vi "Excel Data Log 2.vi"(4 "Channel Settings":T9={"Supply Voltage [Vdc]"=14.4, "Max Supply Current [Idc]"=50.0, "Settling Delay"=10.0, "Temp Criteria"=0.0, "Voltage Steps [Vrms]"=[], "User Notes"="", "Config Wave File Path"=path "", "Config Voltage [Vrms]"=0.1, "Channel Configuration List"={"Channel Configuration Cluster"={"Input"=enum."1 AVG", "Enable"=TRUE, "User Notes"="1", "Voltage Range"=15.0, "Current Range"=2.5}, "Channel Configuration Cluster 2"={"Input"=enum."1 AVG", "Enable"=TRUE, "User Notes"="2", "Voltage Range"=15.0, "Current Range"=2.5}, "Channel Configuration Cluster 3"={"Input"=enum."1 AVG", "Enable"=TRUE, "User Notes"="3", "Voltage Range"=15.0, "Current Range"=2.5}, "Channel Configuration Cluster 4"={"Input"=enum."1 AVG", "Enable"=TRUE, "User Notes"="4", "Voltage Range"=15.0, "Current Range"=2.5}, "Channel Configuration Cluster 5"={"Input"=enum."1", "Enable"=TRUE, "User Notes"="5", "Voltage Range"=15.0, "Current Range"=2.5}, "Channel Configuration Cluster 6"={"Input"=enum."1", "Enable"=TRUE, "User Notes"="6", "Voltage Range"=15.0, "Current Range"=2.5}, "Channel Configuration Cluster 7"={"Input"=enum."1", "Enable"=TRUE, "User Notes"="7", "Voltage Range"=15.0, "Current Range"=2.5}, "Channel Configuration Cluster 8"={"Input"=enum."1", "Enable"=TRUE, "User Notes"="8", "Voltage Range"=15.0, "Current Range"=2.5}, "Channel Configuration Cluster 9"={"Input"=enum."1", "Enable"=TRUE, "User Notes"="9", "Voltage Range"=15.0, "Current Range"=2.5}, "Channel Configuration Cluster 10"={"Input"=enum."2 AVG", "Enable"=TRUE, "User Notes"="10", "Voltage Range"=15.0, "Current Range"=2.5}, "Channel Configuration Cluster 11"={"Input"=enum."2 AVG", "Enable"=TRUE, "User Notes"="11", "Voltage Range"=15.0, "Current Range"=2.5}, "Channel Configuration Cluster 12"={"Input"=enum."2 AVG", "Enable"=TRUE, "User Notes"="12", "Voltage Range"=15.0, "Current Range"=2.5}, "Channel Configuration Cluster 13"={"Input"=enum."2 AVG", "Enable"=TRUE, "User Notes"="13", "Voltage Range"=15.0, "Current Range"=2.5}, "Channel Configuration Cluster 14"={"Input"=enum."2", "Enable"=TRUE, "User Notes"="14", "Voltage Range"=15.0, "Current Range"=2.5}, "Channel Configuration Cluster 15"={"Input"=enum."2", "Enable"=TRUE, "User Notes"="15", "Voltage Range"=15.0, "Current Range"=2.5}, "Channel Configuration Cluster 16"={"Input"=enum."2", "Enable"=TRUE, "User Notes"="16", "Voltage Range"=15.0, "Current Range"=2.5}, "Channel Configuration Cluster 17"={"Input"=enum."2", "Enable"=TRUE, "User Notes"="17", "Voltage Range"=15.0, "Current Range"=2.5}}, "User Gains"={"Gain 1"=12.0, "Gain 2"=11.9, "Gain 3"=0.0, "Gain 4"=0.0, "Gain 5"=0.0, "Gain 6"=0.0}, "Gains"={"Gain 1"=11.908530403349321, "Gain 2"=11.85949105887029, "Gain 3"=0.0, "Gain 4"=0.0, "Gain 5"=0.0, "Gain 6"=0.0}, "Gain Array"={"Gain 1"=11.948064032758305, "Gain 2"=11.797736859280617, "Gain 3"=11.962639910718805, "Gain 4"=11.924703126556764, "Gain 5"=11.642892109168656, "Gain 6"=11.458169944769443, "Gain 7"=11.65709969408898, "Gain 8"=11.754705913936172, "Gain 9"=11.848154878633066, "Gain 10"=11.818689497840571, "Gain 11"=11.899914309524277, "Gain 12"=11.77881456393431, "Gain 13"=11.93961179471489, "Gain 14"=11.746688316913492, "Gain 15"=11.861889454079613, "Gain 16"=11.852640030144613, "Gain 17"=11.690623229258875}, "Wave File Path 1"=path "C:/Users/gm8988/Desktop/Data Log", "Wave File Path 2"=path "", "Wave File Path 3"=path "", "Wave File Path 4"=path "", "Range"=FALSE, "CF"=FALSE} {"Gain Array"."Gain 17" format="%.2f"; "Gain Array"."Gain 16" format="%.2f"; "Gain Array"."Gain 15" format="%.2f"; "Gain Array"."Gain 14" format="%.2f"; "Gain Array"."Gain 13" format="%.2f"; "Gain Array"."Gain 12" format="%.2f"; "Gain Array"."Gain 11" format="%.2f"; "Gain Array"."Gain 10" format="%.2f"; "Gain Array"."Gain 9" format="%.2f"; "Gain Array"."Gain 8" format="%.2f"; "Gain Array"."Gain 7" format="%.2f"; "Gain Array"."Gain 6" format="%.2f"; "Gain Array"."Gain 5" format="%.2f"; "Gain Array"."Gain 4" format="%.2f"; "Gain Array"."Gain 3" format="%.2f"; "Gain Array"."Gain 2" format="%.2f"; "Gain Array"."Gain 1" format="%.2f"; "Gains"."Gain 6" format="%.2f"; "Gains"."Gain 5" format="%.2f"; "Gains"."Gain 4" format="%.2f"; "Gains"."Gain 3" format="%.2f"; "Gains"."Gain 2" format="%.2f"; "Gains"."Gain 1" format="%.2f"; "User Gains"."Gain 6" format="%.2f"; "User Gains"."Gain 5" format="%.2f"; "User Gains"."Gain 4" format="%.2f"; "User Gains"."Gain 3" format="%.2f"; "User Gains"."Gain 2" format="%.2f"; "User Gains"."Gain 1" format="%.2f"; "Channel Configuration List"."Channel Configuration Cluster 17"."Current Range" items=["1 <500m>"=0.5, "2 <1>"=1.0, "5 <2.5>"=2.5, "10 <5>"=5.0, "20 <10>"=10.0, "50 <25>"=25.0]; "Channel Configuration List"."Channel Configuration Cluster 17"."Voltage Range" items=["1.5 <0.75>"=0.75, "3 <1.5>"=1.5, "6 <3>"=3.0, "10 <5>"=5.0, "15 <7.5>"=7.5, "30 <15>"=15.0, "60 <30>"=30.0, "100 <50>"=50.0, "150 <75>"=75.0, "300 <150>"=150.0, "600 <300>"=300.0, "1000 <500>"=500.0]; "Channel Configuration List"."Channel Configuration Cluster 16"."Current Range" items=["1 <500m>"=0.5, "2 <1>"=1.0, "5 <2.5>"=2.5, "10 <5>"=5.0, "20 <10>"=10.0, "50 <25>"=25.0]; "Channel Configuration List"."Channel Configuration Cluster 16"."Voltage Range" items=["1.5 <0.75>"=0.75, "3 <1.5>"=1.5, "6 <3>"=3.0, "10 <5>"=5.0, "15 <7.5>"=7.5, "30 <15>"=15.0, "60 <30>"=30.0, "100 <50>"=50.0, "150 <75>"=75.0, "300 <150>"=150.0, "600 <300>"=300.0, "1000 <500>"=500.0]; "Channel Configuration List"."Channel Configuration Cluster 15"."Current Range" items=["1 <500m>"=0.5, "2 <1>"=1.0, "5 <2.5>"=2.5, "10 <5>"=5.0, "20 <10>"=10.0, "50 <25>"=25.0]; "Channel Configuration List"."Channel Configuration Cluster 15"."Voltage Range" items=["1.5 <0.75>"=0.75, "3 <1.5>"=1.5, "6 <3>"=3.0, "10 <5>"=5.0, "15 <7.5>"=7.5, "30 <15>"=15.0, "60 <30>"=30.0, "100 <50>"=50.0, "150 <75>"=75.0, "300 <150>"=150.0, "600 <300>"=300.0, "1000 <500>"=500.0]; "Channel Configuration List"."Channel Configuration Cluster 14"."Current Range" items=["1 <500m>"=0.5, "2 <1>"=1.0, "5 <2.5>"=2.5, "10 <5>"=5.0, "20 <10>"=10.0, "50 <25>"=25.0]; "Channel Configuration List"."Channel Configuration Cluster 14"."Voltage Range" items=["1.5 <0.75>"=0.75, "3 <1.5>"=1.5, "6 <3>"=3.0, "10 <5>"=5.0, "15 <7.5>"=7.5, "30 <15>"=15.0, "60 <30>"=30.0, "100 <50>"=50.0, "150 <75>"=75.0, "300 <150>"=150.0, "600 <300>"=300.0, "1000 <500>"=500.0]; "Channel Configuration List"."Channel Configuration Cluster 13"."Current Range" items=["1 <500m>"=0.5, "2 <1>"=1.0, "5 <2.5>"=2.5, "10 <5>"=5.0, "20 <10>"=10.0, "50 <25>"=25.0]; "Channel Configuration List"."Channel Configuration Cluster 13"."Voltage Range" items=["1.5 <0.75>"=0.75, "3 <1.5>"=1.5, "6 <3>"=3.0, "10 <5>"=5.0, "15 <7.5>"=7.5, "30 <15>"=15.0, "60 <30>"=30.0, "100 <50>"=50.0, "150 <75>"=75.0, "300 <150>"=150.0, "600 <300>"=300.0, "1000 <500>"=500.0]; "Channel Configuration List"."Channel Configuration Cluster 12"."Current Range" items=["1 <500m>"=0.5, "2 <1>"=1.0, "5 <2.5>"=2.5, "10 <5>"=5.0, "20 <10>"=10.0, "50 <25>"=25.0]; "Channel Configuration List"."Channel Configuration Cluster 12"."Voltage Range" items=["1.5 <0.75>"=0.75, "3 <1.5>"=1.5, "6 <3>"=3.0, "10 <5>"=5.0, "15 <7.5>"=7.5, "30 <15>"=15.0, "60 <30>"=30.0, "100 <50>"=50.0, "150 <75>"=75.0, "300 <150>"=150.0, "600 <300>"=300.0, "1000 <500>"=500.0]; "Channel Configuration List"."Channel Configuration Cluster 11"."Current Range" items=["1 <500m>"=0.5, "2 <1>"=1.0, "5 <2.5>"=2.5, "10 <5>"=5.0, "20 <10>"=10.0, "50 <25>"=25.0]; "Channel Configuration List"."Channel Configuration Cluster 11"."Voltage Range" items=["1.5 <0.75>"=0.75, "3 <1.5>"=1.5, "6 <3>"=3.0, "10 <5>"=5.0, "15 <7.5>"=7.5, "30 <15>"=15.0, "60 <30>"=30.0, "100 <50>"=50.0, "150 <75>"=75.0, "300 <150>"=150.0, "600 <300>"=300.0, "1000 <500>"=500.0]; "Channel Configuration List"."Channel Configuration Cluster 10"."Current Range" items=["1 <500m>"=0.5, "2 <1>"=1.0, "5 <2.5>"=2.5, "10 <5>"=5.0, "20 <10>"=10.0, "50 <25>"=25.0]; "Channel Configuration List"."Channel Configuration Cluster 10"."Voltage Range" items=["1.5 <0.75>"=0.75, "3 <1.5>"=1.5, "6 <3>"=3.0, "10 <5>"=5.0, "15 <7.5>"=7.5, "30 <15>"=15.0, "60 <30>"=30.0, "100 <50>"=50.0, "150 <75>"=75.0, "300 <150>"=150.0, "600 <300>"=300.0, "1000 <500>"=500.0]; "Channel Configuration List"."Channel Configuration Cluster 9"."Voltage Range" items=["1.5 <0.75>"=0.75, "3 <1.5>"=1.5, "6 <3>"=3.0, "10 <5>"=5.0, "15 <7.5>"=7.5, "30 <15>"=15.0, "60 <30>"=30.0, "100 <50>"=50.0, "150 <75>"=75.0, "300 <150>"=150.0, "600 <300>"=300.0, "1000 <500>"=500.0]; "Channel Configuration List"."Channel Configuration Cluster 9"."Current Range" items=["10m <5m>"=0.005, "20m <10m>"=0.01, "50m <25m>"=0.025, "100m <50m>"=0.05, "200m <100m>"=0.1, "500m <250m>"=0.25, "1 <500m>"=0.5, "2 <1>"=1.0, "5 <2.5>"=2.5]; "Channel Configuration List"."Channel Configuration Cluster 8"."Voltage Range" items=["1.5 <0.75>"=0.75, "3 <1.5>"=1.5, "6 <3>"=3.0, "10 <5>"=5.0, "15 <7.5>"=7.5, "30 <15>"=15.0, "60 <30>"=30.0, "100 <50>"=50.0, "150 <75>"=75.0, "300 <150>"=150.0, "600 <300>"=300.0, "1000 <500>"=500.0]; "Channel Configuration List"."Channel Configuration Cluster 8"."Current Range" items=["10m <5m>"=0.005, "20m <10m>"=0.01, "50m <25m>"=0.025, "100m <50m>"=0.05, "200m <100m>"=0.1, "500m <250m>"=0.25, "1 <500m>"=0.5, "2 <1>"=1.0, "5 <2.5>"=2.5]; "Channel Configuration List"."Channel Configuration Cluster 7"."Voltage Range" items=["1.5 <0.75>"=0.75, "3 <1.5>"=1.5, "6 <3>"=3.0, "10 <5>"=5.0, "15 <7.5>"=7.5, "30 <15>"=15.0, "60 <30>"=30.0, "100 <50>"=50.0, "150 <75>"=75.0, "300 <150>"=150.0, "600 <300>"=300.0, "1000 <500>"=500.0]; "Channel Configuration List"."Channel Configuration Cluster 7"."Current Range" items=["10m <5m>"=0.005, "20m <10m>"=0.01, "50m <25m>"=0.025, "100m <50m>"=0.05, "200m <100m>"=0.1, "500m <250m>"=0.25, "1 <500m>"=0.5, "2 <1>"=1.0, "5 <2.5>"=2.5]; "Channel Configuration List"."Channel Configuration Cluster 6"."Voltage Range" items=["1.5 <0.75>"=0.75, "3 <1.5>"=1.5, "6 <3>"=3.0, "10 <5>"=5.0, "15 <7.5>"=7.5, "30 <15>"=15.0, "60 <30>"=30.0, "100 <50>"=50.0, "150 <75>"=75.0, "300 <150>"=150.0, "600 <300>"=300.0, "1000 <500>"=500.0]; "Channel Configuration List"."Channel Configuration Cluster 6"."Current Range" items=["10m <5m>"=0.005, "20m <10m>"=0.01, "50m <25m>"=0.025, "100m <50m>"=0.05, "200m <100m>"=0.1, "500m <250m>"=0.25, "1 <500m>"=0.5, "2 <1>"=1.0, "5 <2.5>"=2.5]; "Channel Configuration List"."Channel Configuration Cluster 5"."Voltage Range" items=["1.5 <0.75>"=0.75, "3 <1.5>"=1.5, "6 <3>"=3.0, "10 <5>"=5.0, "15 <7.5>"=7.5, "30 <15>"=15.0, "60 <30>"=30.0, "100 <50>"=50.0, "150 <75>"=75.0, "300 <150>"=150.0, "600 <300>"=300.0, "1000 <500>"=500.0]; "Channel Configuration List"."Channel Configuration Cluster 5"."Current Range" items=["10m <5m>"=0.005, "20m <10m>"=0.01, "50m <25m>"=0.025, "100m <50m>"=0.05, "200m <100m>"=0.1, "500m <250m>"=0.25, "1 <500m>"=0.5, "2 <1>"=1.0, "5 <2.5>"=2.5]; "Channel Configuration List"."Channel Configuration Cluster 4"."Voltage Range" items=["1.5 <0.75>"=0.75, "3 <1.5>"=1.5, "6 <3>"=3.0, "10 <5>"=5.0, "15 <7.5>"=7.5, "30 <15>"=15.0, "60 <30>"=30.0, "100 <50>"=50.0, "150 <75>"=75.0, "300 <150>"=150.0, "600 <300>"=300.0, "1000 <500>"=500.0]; "Channel Configuration List"."Channel Configuration Cluster 4"."Current Range" items=["10m <5m>"=0.005, "20m <10m>"=0.01, "50m <25m>"=0.025, "100m <50m>"=0.05, "200m <100m>"=0.1, "500m <250m>"=0.25, "1 <500m>"=0.5, "2 <1>"=1.0, "5 <2.5>"=2.5]; "Channel Configuration List"."Channel Configuration Cluster 3"."Voltage Range" items=["1.5 <0.75>"=0.75, "3 <1.5>"=1.5, "6 <3>"=3.0, "10 <5>"=5.0, "15 <7.5>"=7.5, "30 <15>"=15.0, "60 <30>"=30.0, "100 <50>"=50.0, "150 <75>"=75.0, "300 <150>"=150.0, "600 <300>"=300.0, "1000 <500>"=500.0]; "Channel Configuration List"."Channel Configuration Cluster 3"."Current Range" items=["10m <5m>"=0.005, "20m <10m>"=0.01, "50m <25m>"=0.025, "100m <50m>"=0.05, "200m <100m>"=0.1, "500m <250m>"=0.25, "1 <500m>"=0.5, "2 <1>"=1.0, "5 <2.5>"=2.5]; "Channel Configuration List"."Channel Configuration Cluster 2"."Voltage Range" items=["1.5 <0.75>"=0.75, "3 <1.5>"=1.5, "6 <3>"=3.0, "10 <5>"=5.0, "15 <7.5>"=7.5, "30 <15>"=15.0, "60 <30>"=30.0, "100 <50>"=50.0, "150 <75>"=75.0, "300 <150>"=150.0, "600 <300>"=300.0, "1000 <500>"=500.0]; "Channel Configuration List"."Channel Configuration Cluster 2"."Current Range" items=["10m <5m>"=0.005, "20m <10m>"=0.01, "50m <25m>"=0.025, "100m <50m>"=0.05, "200m <100m>"=0.1, "500m <250m>"=0.25, "1 <500m>"=0.5, "2 <1>"=1.0, "5 <2.5>"=2.5]; "Channel Configuration List"."Channel Configuration Cluster"."Voltage Range" items=["1.5 <0.75>"=0.75, "3 <1.5>"=1.5, "6 <3>"=3.0, "10 <5>"=5.0, "15 <7.5>"=7.5, "30 <15>"=15.0, "60 <30>"=30.0, "100 <50>"=50.0, "150 <75>"=75.0, "300 <150>"=150.0, "600 <300>"=300.0, "1000 <500>"=500.0]; "Channel Configuration List"."Channel Configuration Cluster"."Current Range" items=["10m <5m>"=0.005, "20m <10m>"=0.01, "50m <25m>"=0.025, "100m <50m>"=0.05, "200m <100m>"=0.1, "500m <250m>"=0.25, "1 <500m>"=0.5, "2 <1>"=1.0, "5 <2.5>"=2.5]; "Settling Delay" min=0.0 format="%<%H:%M:%S>t"}, 5 "JPEG2 Path":path, 6 "Cancel":bool, 7 "JPEG1 Path":path, 8 "error in":errorcluster, 10 "Datalog Cluster Array":T1 {"WT1800 Averages"."Vrms" format="%.3f"; "WT1800 Averages"."Irms" format="%.3f"; "WT1800 Averages"."Power" format="%.3f"; "WT1800 Averages"."Vpkpk" format="%.3f"; "WT1800 Averages"."Ipkpk" format="%.3f"; "WT1800 Measurements"."Vrms" format="%.3f"; "WT1800 Measurements"."Irms" format="%.3f"; "WT1800 Measurements"."Power" format="%.3f"; "WT1800 Measurements"."Vpkpk" format="%.3f"; "WT1800 Measurements"."Ipkpk" format="%.3f"; "DSA Averages"."Vrms" format="%.3f"; "DSA Averages"."Vdc" format="%.3f"; "DSA Averages"."Vpk+" format="%.3f"; "DSA Averages"."Vpk-" format="%.3f"; "DSA Averages"."Vpkpk" format="%.3f"; "DSA Measurements"."Vrms" format="%.3f"; "DSA Measurements"."Vdc" format="%.3f"; "DSA Measurements"."Vpk+" format="%.3f"; "DSA Measurements"."Vpk-" format="%.3f"; "DSA Measurements"."Vpkpk" format="%.3f"}, 11 "Template Path":path) -> (0 "error out":errorcluster)   [LabVIEW 2021]
uses:
  Datalog Controls/Select_Data.ctl
  Controls/Settings Control.ctl
  Controls/Channel Configuration List.ctl
  Controls/Channel Configuration Cluster.ctl
  Controls/Channel Configuration Cluster High Current.ctl
  Controls/Gain Averages.ctl
  Controls/Gain Array.ctl
  Controls/Datalog Cluster Array.ctl
  Controls/Datalog Bundle Control.ctl
  Controls/WT1800 Functions.ctl
  Controls/WT1800 Measurements.ctl
  Controls/WT1800 Readings.ctl
  Controls/DSA Functions.ctl
  Controls/DSA Measurements.ctl
  Controls/DSA Readings.ctl
  Datalog Controls/States.ctl
  Datalog Controls/Data.ctl
  <vilib>/Utility/NIReport.llb/NI_report.lvclass
  <vilib>/Utility/miscctls.llb/LVPointTypeDef.ctl
  <vilib>/Utility/error.llb/DialogType.ctl
panel:
  out "Time Taken (Seconds)":u32
  in  "Generate":bool
  in  "Manual Select":bool
  in  "Select All":bool=TRUE
  in  "Select Data":T15={"Vrms Data"=TRUE, "Vpkpk Data"=TRUE, "Irms Data"=TRUE, "Power Data"=TRUE, "Ipkpk Data"=TRUE, "Temp Data"=TRUE}
  in  "Detailed Report":bool=TRUE
  in  "Stop":bool
  in  "Summary Report":bool
  # "Ver 1.2.1"
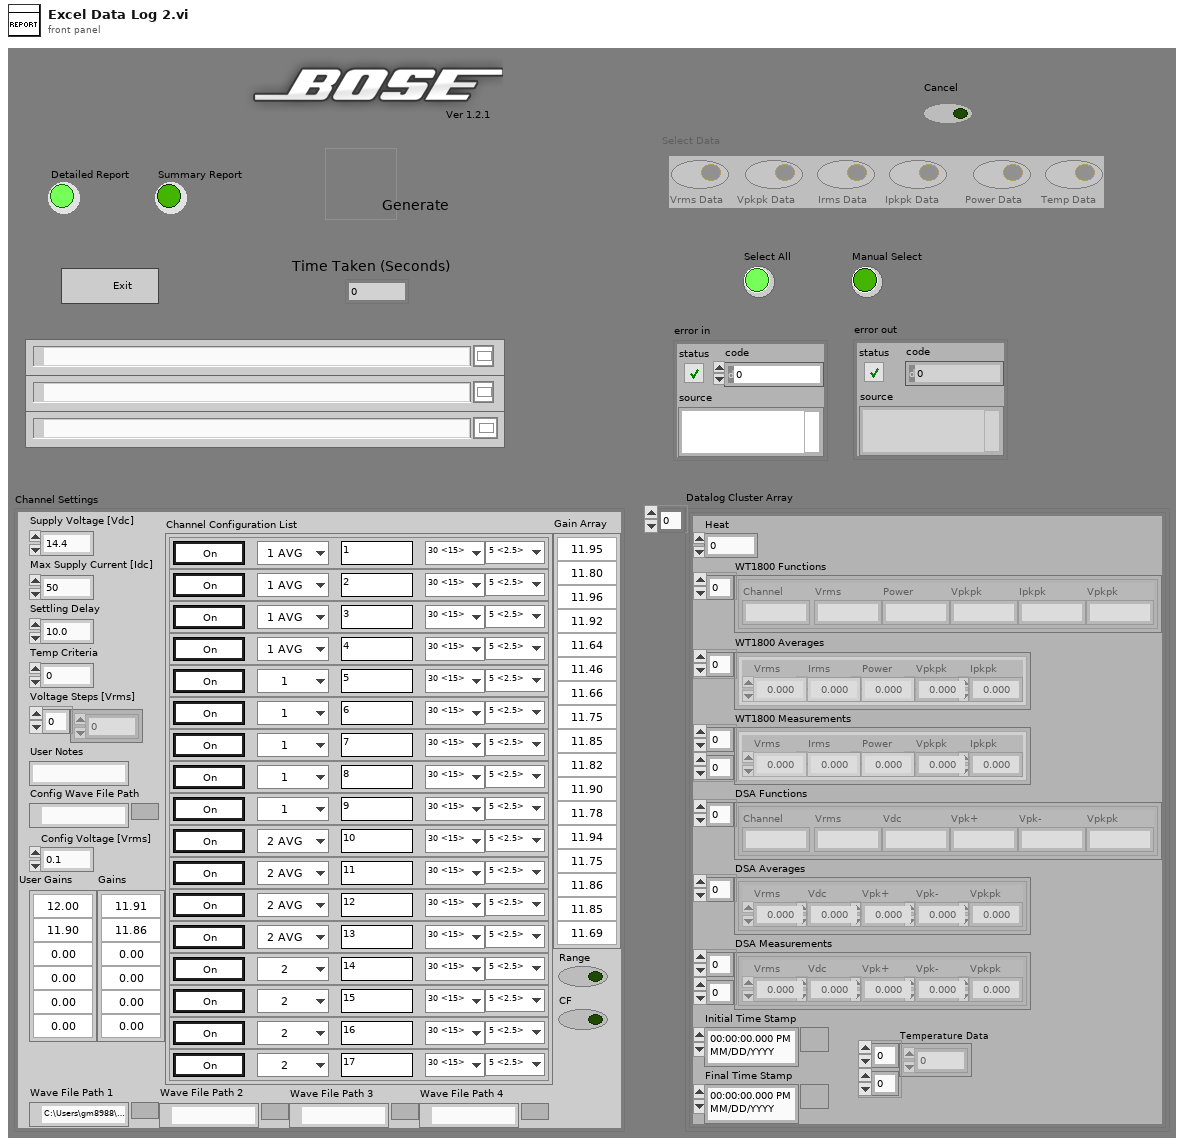
[diagram p1: front panel]
types:
  T1 = typedef "Datalog Cluster Array.ctl" = T2[]
  T2 = typedef "Datalog Bundle Control.ctl" = cluster{"Heat":dbl, "WT1800 Functions":T3, "WT1800 Averages":T4, "WT1800 Measurements":T5[][], "DSA Functions":T6, "DSA Averages":T7, "DSA Measurements":T8[][], "Initial Time Stamp":timestamp, "Final Time Stamp":timestamp, "Temperature Data":sgl[][]}
  T3 = typedef "WT1800 Functions.ctl" = cluster{"Channel":string, "Vrms":string, "Power":string, "Vpkpk":string, "Ipkpk":string, "Vpkpk":string}[]
  T4 = typedef "WT1800 Measurements.ctl" = T5[]
  T5 = typedef "WT1800 Readings.ctl" = cluster{"Vrms":sgl, "Irms":sgl, "Power":sgl, "Vpkpk":sgl, "Ipkpk":sgl}
  T6 = typedef "DSA Functions.ctl" = cluster{"Channel":string, "Vrms":string, "Vdc":string, "Vpk+":string, "Vpk-":string, "Vpkpk":string}[]
  T7 = typedef "DSA Measurements.ctl" = T8[]
  T8 = typedef "DSA Readings.ctl" = cluster{"Vrms":sgl, "Vdc":sgl, "Vpk+":sgl, "Vpk-":sgl, "Vpkpk":sgl}
  T9 = typedef "Settings Control.ctl" = cluster{"Supply Voltage [Vdc]":sgl, "Max Supply Current [Idc]":sgl, "Settling Delay":dbl, "Temp Criteria":sgl, "Voltage Steps [Vrms]":sgl[], "User Notes":string, "Config Wave File Path":path, "Config Voltage [Vrms]":sgl, "Channel Configuration List":T10, "User Gains":T13, "Gains":T13, "Gain Array":T14, "Wave File Path 1":path, "Wave File Path 2":path, "Wave File Path 3":path, "Wave File Path 4":path, "Range":bool, "CF":bool}
  T10 = typedef "Channel Configuration List.ctl" = cluster{"Channel Configuration Cluster":T11, "Channel Configuration Cluster 2":T11, "Channel Configuration Cluster 3":T11, "Channel Configuration Cluster 4":T11, "Channel Configuration Cluster 5":T11, "Channel Configuration Cluster 6":T11, "Channel Configuration Cluster 7":T11, "Channel Configuration Cluster 8":T11, "Channel Configuration Cluster 9":T11, "Channel Configuration Cluster 10":T12, "Channel Configuration Cluster 11":T12, "Channel Configuration Cluster 12":T12, "Channel Configuration Cluster 13":T12, "Channel Configuration Cluster 14":T12, "Channel Configuration Cluster 15":T12, "Channel Configuration Cluster 16":T12, "Channel Configuration Cluster 17":T12}
  T11 = typedef "Channel Configuration Cluster.ctl" = cluster{"Input":enum16{"---", "1", "1 AVG", "2", "2 AVG", "3", "3 AVG", "4", "4 AVG"}, "Enable":bool, "User Notes":string, "Voltage Range":dbl, "Current Range":dbl}
  T12 = typedef "Channel Configuration Cluster High Current.ctl" = cluster{"Input":enum16{"---", "1", "1 AVG", "2", "2 AVG", "3", "3 AVG", "4", "4 AVG"}, "Enable":bool, "User Notes":string, "Voltage Range":dbl, "Current Range":dbl}
  T13 = typedef "Gain Averages.ctl" = cluster{"Gain 1":dbl, "Gain 2":dbl, "Gain 3":dbl, "Gain 4":dbl, "Gain 5":dbl, "Gain 6":dbl}
  T14 = typedef "Gain Array.ctl" = cluster{"Gain 1":dbl, "Gain 2":dbl, "Gain 3":dbl, "Gain 4":dbl, "Gain 5":dbl, "Gain 6":dbl, "Gain 7":dbl, "Gain 8":dbl, "Gain 9":dbl, "Gain 10":dbl, "Gain 11":dbl, "Gain 12":dbl, "Gain 13":dbl, "Gain 14":dbl, "Gain 15":dbl, "Gain 16":dbl, "Gain 17":dbl}
  T15 = typedef "Select_Data.ctl" = cluster{"Vrms Data":bool, "Vpkpk Data":bool, "Irms Data":bool, "Power Data":bool, "Ipkpk Data":bool, "Temp Data":bool}
  T16 = typedef "Data.ctl" = cluster{"Input Data 1D":T1, "Channel Settings":T9, "Select Data":T15, "Detailed Report ?":bool, "Path Settings:":cluster{"Template Path ":path, "Report Path":path, "JPEG1 Path ":path, "JPEG2 Path":path}, "Vrms_Sheet":string[][], "Irms_Sheet":string[][], "Power_Sheet":string[][], "Vpk_Sheet":string[][], "Ipk_Sheet":string[][], "Vrms_Avg":string[][], "Irms_Avg":string[][], "Power_Avg":string[][], "Vpk_Avg":string[][], "Ipk_Avg":string[][], "Report_Ref":refnum<class "NI_report.lvclass">, "User Name":string, "Temp_Sheet":string[][]}
  T17 = typedef "States.ctl" = enum16{"Initialize", "Poll", "Generate Report", "Error", "Exit"}
  T18 = typedef "LVPointTypeDef.ctl" = cluster{"Horizontal":i16, "Vertical":i16}
  T19 = enum8{"Enabled", "Disabled", "Disabled and Grayed Out"}
  T20 = typedef "DialogType.ctl" = u16
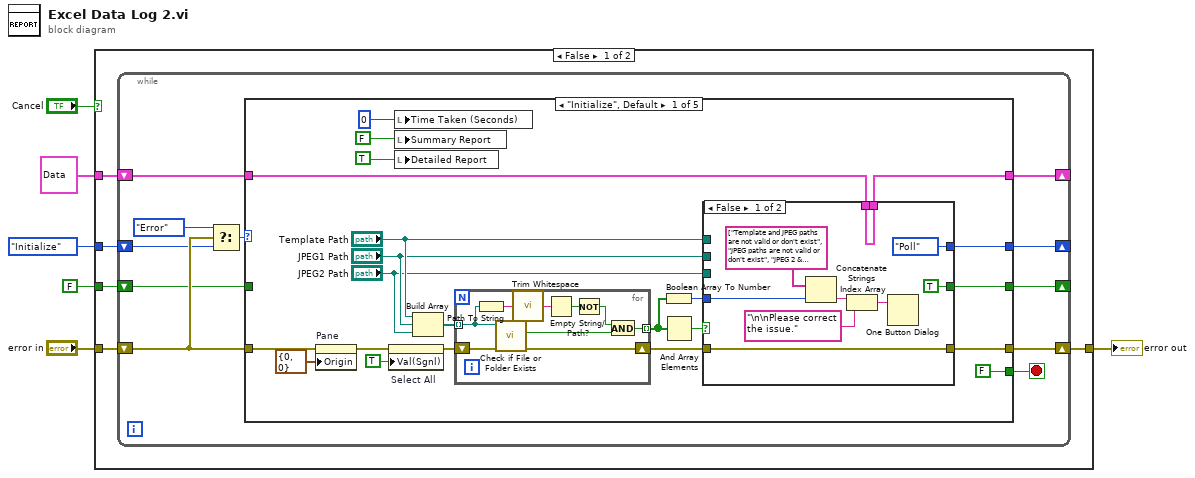
[diagram p0: block diagram]
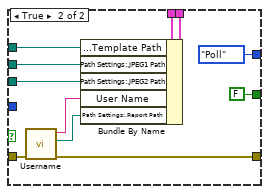
[diagram p2: hidden frame]
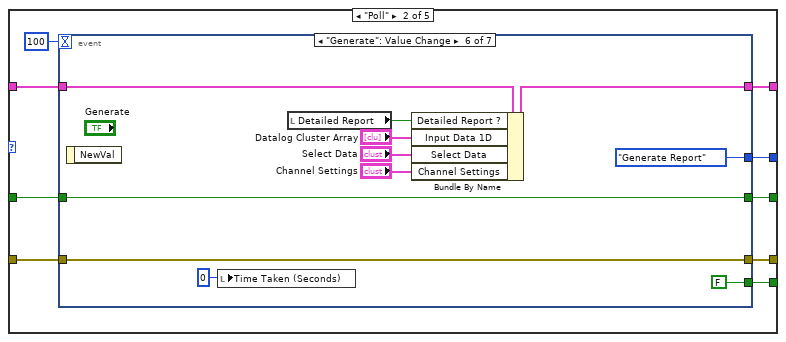
[diagram p3: hidden frame]
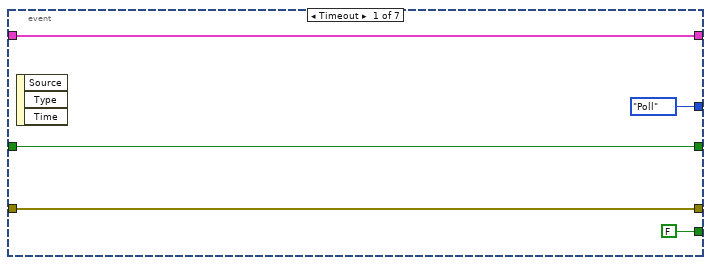
[diagram p4: hidden frame]
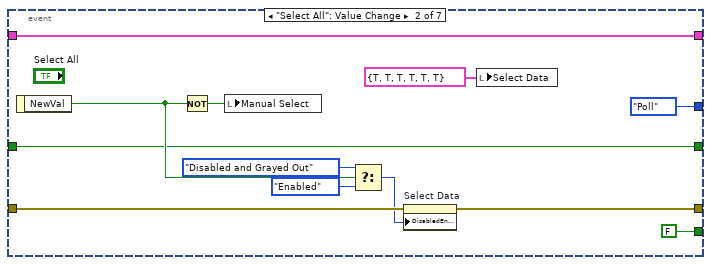
[diagram p5: hidden frame]
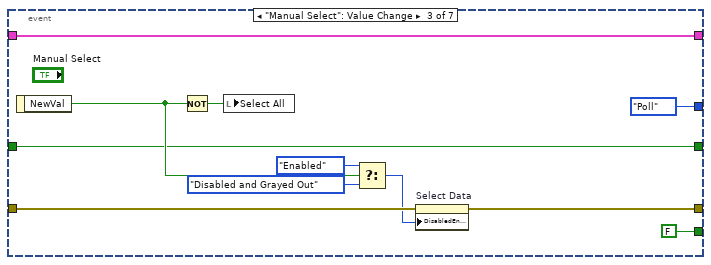
[diagram p6: hidden frame]
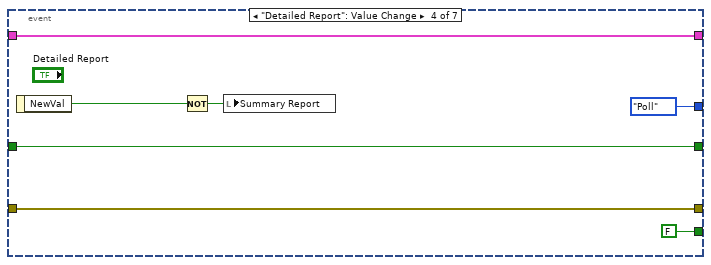
[diagram p7: hidden frame]
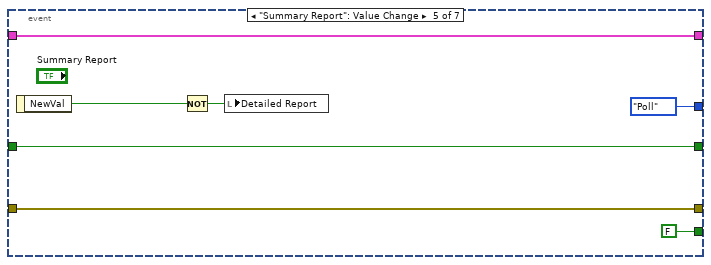
[diagram p8: hidden frame]
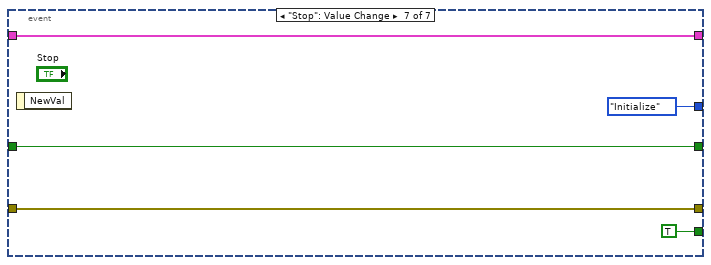
[diagram p9: hidden frame]
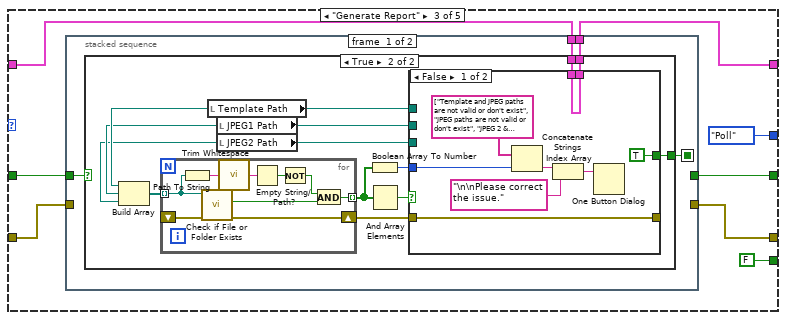
[diagram p10: hidden frame]
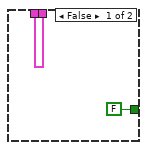
[diagram p11: hidden frame]
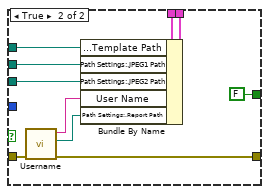
[diagram p12: hidden frame]
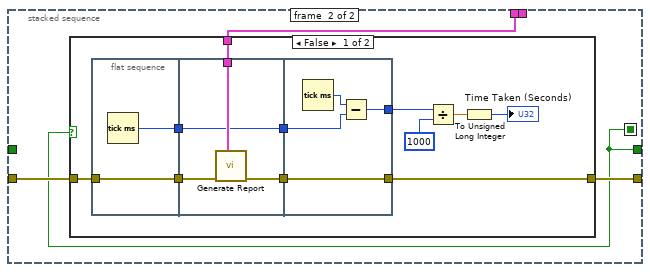
[diagram p13: hidden frame]
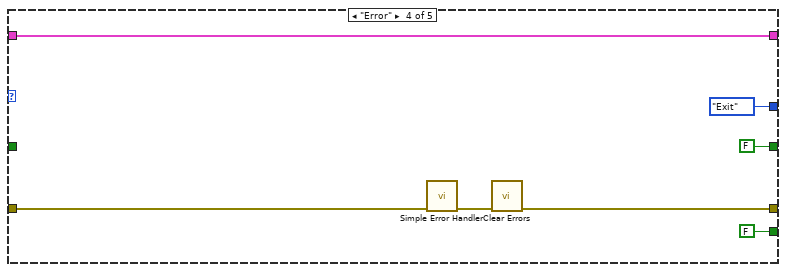
[diagram p15: hidden frame]
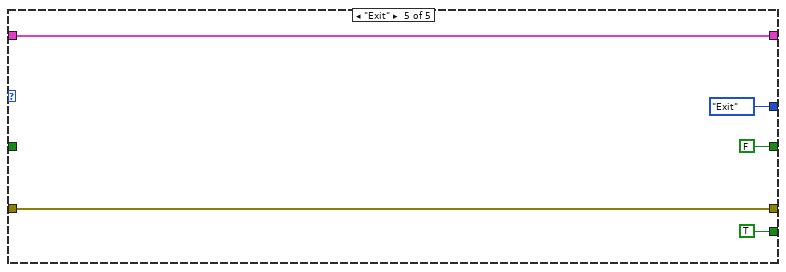
[diagram p16: hidden frame]
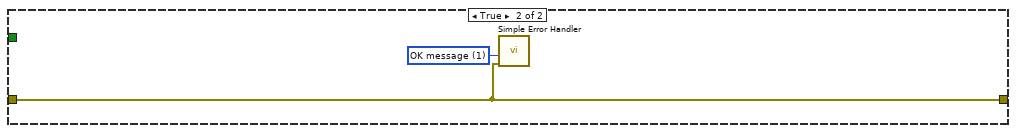
[diagram p17: hidden frame]
diagram:
  n1 = case shown="False" "Cancel" {
    tunnel: States."Initialize" -> [w11 _]
    tunnel: T16 {"Input Data 1D"=[], "Channel Settings"={"Supply Voltage [Vdc]"=0.0, "Max Supply Current [Idc]"=0.0, "Settling Delay"=0.0, "Temp Criteria"=0.0, "Voltage Steps [Vrms]"=[0.0, 0.25, 0.5, 1.0, 1.95, 3.0, 3.9, 5.5], "User Notes"="", "Config Wave File Path"=path "C:/ASD Power Point Beta 32J/Waveforms/150HzSine5Second.wav", "Config Voltage [Vrms]"=0.0, "Channel Configuration List"={"Channel Configuration Cluster"={"Input"=enum."---", "Enable"=FALSE, "User Notes"="", "Voltage Range"=0.0, "Current Range"=2.5}, "Channel Configuration Cluster 2"={"Input"=enum."---", "Enable"=FALSE, "User Notes"="", "Voltage Range"=0.0, "Current Range"=2.5}, "Channel Configuration Cluster 3"={"Input"=enum."---", "Enable"=FALSE, "User Notes"="", "Voltage Range"=0.0, "Current Range"=2.5}, "Channel Configuration Cluster 4"={"Input"=enum."---", "Enable"=FALSE, "User Notes"="", "Voltage Range"=0.0, "Current Range"=2.5}, "Channel Configuration Cluster 5"={"Input"=enum."---", "Enable"=FALSE, "User Notes"="", "Voltage Range"=0.0, "Current Range"=2.5}, "Channel Configuration Cluster 6"={"Input"=enum."---", "Enable"=FALSE, "User Notes"="", "Voltage Range"=0.0, "Current Range"=2.5}, "Channel Configuration Cluster 7"={"Input"=enum."---", "Enable"=FALSE, "User Notes"="", "Voltage Range"=0.0, "Current Range"=2.5}, "Channel Configuration Cluster 8"={"Input"=enum."---", "Enable"=FALSE, "User Notes"="", "Voltage Range"=0.0, "Current Range"=2.5}, "Channel Configuration Cluster 9"={"Input"=enum."---", "Enable"=FALSE, "User Notes"="", "Voltage Range"=0.0, "Current Range"=2.5}, "Channel Configuration Cluster 10"={"Input"=enum."---", "Enable"=FALSE, "User Notes"="", "Voltage Range"=0.0, "Current Range"=2.5}, "Channel Configuration Cluster 11"={"Input"=enum."---", "Enable"=FALSE, "User Notes"="", "Voltage Range"=0.0, "Current Range"=2.5}, "Channel Configuration Cluster 12"={"Input"=enum."---", "Enable"=FALSE, "User Notes"="", "Voltage Range"=0.0, "Current Range"=2.5}, "Channel Configuration Cluster 13"={"Input"=enum."---", "Enable"=FALSE, "User Notes"="", "Voltage Range"=0.0, "Current Range"=2.5}, "Channel Configuration Cluster 14"={"Input"=enum."---", "Enable"=FALSE, "User Notes"="", "Voltage Range"=0.0, "Current Range"=2.5}, "Channel Configuration Cluster 15"={"Input"=enum."---", "Enable"=FALSE, "User Notes"="", "Voltage Range"=0.0, "Current Range"=2.5}, "Channel Configuration Cluster 16"={"Input"=enum."---", "Enable"=FALSE, "User Notes"="", "Voltage Range"=0.0, "Current Range"=2.5}, "Channel Configuration Cluster 17"={"Input"=enum."---", "Enable"=FALSE, "User Notes"="", "Voltage Range"=0.0, "Current Range"=2.5}}, "User Gains"={"Gain 1"=0.0, "Gain 2"=0.0, "Gain 3"=0.0, "Gain 4"=0.0, "Gain 5"=0.0, "Gain 6"=0.0}, "Gains"={"Gain 1"=0.0, "Gain 2"=0.0, "Gain 3"=0.0, "Gain 4"=0.0, "Gain 5"=0.0, "Gain 6"=0.0}, "Gain Array"={"Gain 1"=0.0, "Gain 2"=0.0, "Gain 3"=0.0, "Gain 4"=0.0, "Gain 5"=0.0, "Gain 6"=0.0, "Gain 7"=0.0, "Gain 8"=0.0, "Gain 9"=0.0, "Gain 10"=0.0, "Gain 11"=0.0, "Gain 12"=0.0, "Gain 13"=0.0, "Gain 14"=0.0, "Gain 15"=0.0, "Gain 16"=0.0, "Gain 17"=0.0}, "Wave File Path 1"=path "", "Wave File Path 2"=path "", "Wave File Path 3"=path "", "Wave File Path 4"=path "", "Range"=FALSE, "CF"=FALSE}, "Select Data"={"Vrms Data"=FALSE, "Vpkpk Data"=FALSE, "Irms Data"=FALSE, "Power Data"=FALSE, "Ipkpk Data"=FALSE, "Temp Data"=FALSE}, "Detailed Report ?"=FALSE, "Path Settings:"={"Template Path "=path "E:/L&T Projects/Bose ASD/Excel Template/ASD Template.xltx", "Report Path"=path "E:/L&T Projects/Bose ASD/excel Reports", "JPEG1 Path "=path "C:/Users/Public/Pictures/Sample Pictures/Hydrangeas.jpg", "JPEG2 Path"=path "C:/Users/Public/Pictures/Sample Pictures/Lighthouse.jpg"}, "Vrms_Sheet"=[], "Irms_Sheet"=[], "Power_Sheet"=[], "Vpk_Sheet"=[], "Ipk_Sheet"=[], "Vrms_Avg"=[], "Irms_Avg"=[], "Power_Avg"=[], "Vpk_Avg"=[], "Ipk_Avg"=[], "Report_Ref"=refnum, "User Name"="", "Temp_Sheet"=[]} -> [w10 _]
    tunnel: "error in" -> [w9 w232]
    tunnel: [w8 w232] -> w4
    tunnel: FALSE -> [w7 _]
    frame False {
      n2 = while {
        shift-right: [w18] -> _
        shift-left: w11 -> [w15]
        shift-right: [w21] -> _
        shift-left: w10 -> [w22]
        shift-right: [w19] -> w8
        shift-left: w9 -> [w17]
        shift-right: [w13] -> _
        shift-left: w7 -> [w12]
        stop <- w20 stop-if-true
        n3 = Select(t=States."Error", s=w17, f=w15) -> (s? t:f=w14:T17)
        n4 = case shown="\"Initialize\", Default" w14 {
          tunnel: w22 -> [w38 w81 w146 w224 w228]
          tunnel: [w37 w82 w145 w224 w228] -> w21
          tunnel: [FALSE w80 FALSE FALSE TRUE] -> w20
          tunnel: w17 -> [w36 w79 w143 w222 w230]
          tunnel: [w24 w78 w142 w220 w230] -> w19
          tunnel: [w33 w77 States."Poll" States."Exit" States."Exit"] -> w18
          tunnel: [w23 w75 w141 FALSE FALSE] -> w13
          tunnel: w12 -> [_ w74 w144 _ _]
          frame "Initialize", Default {
            n5 = property on="Pane" class="Pane"(error in=w36, "Origin"=T18 {"Horizontal"=0, "Vertical"=0}) -> (error out=w26:errorcluster)  [unwired: 1 in, 1 out]
            n6 = property on="Select All" class="Bool (strict)"(error in=w26, "Val(Sgnl)"=TRUE ("Value (Signaling)")) -> (error out=w25:errorcluster)  [unwired: 1 in, 1 out]
            n7 = local write "Time Taken (Seconds)"(u32 0 ("Time Taken (Second)")) -> ()
            n8 = local write "Summary Report"(FALSE ("Summary Report")) -> ()
            n9 = local write "Detailed Report"(TRUE ("Select All")) -> ()
            n10 = Build Array("Template Path", "JPEG1 Path", "JPEG2 Path") -> (w35:path[])
            n11 = for {
              tunnel: w35 -> [w69] mode=indexing
              tunnel: [w66] -> w31 mode=indexing
              shift-right: [w72] -> w34
              shift-left: w25 -> [w73]
              n12 = Path To String(path=w69) -> (string=w70:string)
              n13 = call <vilib>:"Check if File or Folder Exists.vi"("error in (no error)"=w73, "path"=w69) -> ("error out"=w72:errorcluster, "file or folder exists?"=w68:bool)  [unwired: 7 in, 1 out]
              n14 = call <vilib>:"Trim Whitespace.vi"("string"=w70) -> ("trimmed string"=w71:string)  [unwired: 1 in]
              n15 = Empty String/Path?(string/path=w71) -> (empty?=w67:bool)
              n16 = Not(x=w67) -> (.not. x?=w65:bool)
              n17 = And(x=w65, y=w68) -> (x .and. y?=w66:bool)
            }
            n18 = Boolean Array To Number(Boolean array=w31) -> (number=w30:u32)
            n19 = And Array Elements(Boolean array=w31) -> (logical AND=w32:bool)
            n20 = case shown="False" w32 {
              tunnel: w38 -> [w49 w64]
              tunnel: [w49 w63] -> w37
              tunnel: [w51 w62] -> w24
              tunnel: w34 -> [w51 w59]
              tunnel: [States."Poll" States."Poll"] -> w33
              tunnel: w30 -> [w52 _]
              tunnel: "Template Path" -> [_ w57]
              tunnel: "JPEG1 Path" -> [_ w56]
              tunnel: "JPEG2 Path" -> [_ w55]
              tunnel: [TRUE FALSE] -> w23
              frame False {
                n21 = Index Array(array=string[] ["Template and JPEG paths are not valid or don't exist", "JPEG paths are not valid or don't exist", "JPEG 2 & Template  paths are not valid", "JPEG 2 path is not valid", "JPEG 1 & Template  paths are not valid", "JPEG 1 path is not valid", "Template path is not valid"], index=w52) -> (element=w47:string)
                n22 = Concatenate Strings(w47, "\n\nPlease correct the issue." ("string")) -> (w46:string)
                n23 = One Button Dialog(message=w46) -> ()  [unwired: 1 in, 1 out]
              }
              frame True {
                n24 = call "Username.vi"("error in"=w59) -> ("error out"=w62:errorcluster, "Report Store Path_Out"=w60:path, "User Name_Out"=w61:string)  [unwired: 8 in]
                n25 = Bundle By Name(cluster=w64, "Path Settings:.Template Path"=w57, "Path Settings:.JPEG1 Path"=w56, "Path Settings:.JPEG2 Path"=w55, "User Name"=w61, "Path Settings:.Report Path"=w60) -> (w63:T16)
              }
            }
          }
          frame "Poll" {
            n26 = event shown="[5] \"Generate\": Value Change" {
              selector: _ -> [_ _ _ _ _ _ _]
              dyn-events: _ -> [_ _ _ _ _ _ _]
              timeout: 100 -> [_ _ _ _ _ _ _]
              tunnel: [w87 w90 w106 w115 w122 w125 w140] -> w82
              tunnel: w81 -> [w87 w90 w106 w115 w122 w126 w140]
              tunnel: [FALSE FALSE FALSE FALSE FALSE FALSE TRUE] -> w80
              tunnel: w79 -> [w84 w97 w108 w112 w119 w134 w137]
              tunnel: [w84 w96 w107 w112 w119 w134 w137] -> w78
              tunnel: [States."Poll" States."Poll" States."Poll" States."Poll" States."Poll" States."Generate Report" States."Initialize"] -> w77
              tunnel: [w83 w88 w100 w111 w118 w131 w136] -> w75
              tunnel: w74 -> [w83 w88 w100 w111 w118 w131 w136]
              event Timeout {
                n27 = event-data() -> ()  [unwired: 1 in, 3 out]
              }
              event "Select All": Value Change {
                n28 = event-data() -> ("NewVal"=w94:bool)  [unwired: 1 in]
                n29 = Not(x=w94) -> (.not. x?=w98:bool)
                n30 = local write "Manual Select"(w98) -> ()
                n31 = Select(t=T19."Disabled and Grayed Out" ("Disabled"), s=w94, f=T19."Enabled") -> (s? t:f=w91:T19)
                n32 = property on="Select Data" class="Clust (strict)"(error in=w97, "DisabledEnum"=w91) -> (error out=w96:errorcluster)  [unwired: 1 in, 1 out]
                n33 = local write "Select Data"(T15 {"Vrms Data"=TRUE, "Vpkpk Data"=TRUE, "Irms Data"=TRUE, "Power Data"=TRUE, "Ipkpk Data"=TRUE, "Temp Data"=TRUE} ("Select Data")) -> ()
              }
              event "Manual Select": Value Change {
                n34 = event-data() -> ("NewVal"=w104:bool)  [unwired: 1 in]
                n35 = Not(x=w104) -> (.not. x?=w109:bool)
                n36 = local write "Select All"(w109) -> ()
                n37 = Select(t=T19."Enabled" ("Disabled"), s=w104, f=T19."Disabled and Grayed Out" ("Disabled")) -> (s? t:f=w101:T19)
                n38 = property on="Select Data" class="Clust (strict)"(error in=w108, "DisabledEnum"=w101) -> (error out=w107:errorcluster)  [unwired: 1 in, 1 out]
              }
              event "Detailed Report": Value Change {
                n39 = event-data() -> ("NewVal"=w113:bool)  [unwired: 1 in]
                n40 = Not(x=w113) -> (.not. x?=w116:bool)
                n41 = local write "Summary Report"(w116) -> ()
              }
              event "Summary Report": Value Change {
                n42 = event-data() -> ("NewVal"=w120:bool)  [unwired: 1 in]
                n43 = Not(x=w120) -> (.not. x?=w123:bool)
                n44 = local write "Detailed Report"(w123) -> ()
              }
              event "Generate": Value Change {
                n45 = event-data() -> ()  [unwired: 1 in, 1 out]
                n46 = local write "Time Taken (Seconds)"(u32 0 ("Numeric")) -> ()
                n47 = local read "Detailed Report"() -> (w130:bool)
                n48 = Bundle By Name(cluster=w126, "Detailed Report ?"=w130, "Input Data 1D"="Datalog Cluster Array", "Select Data"="Select Data", "Channel Settings"="Channel Settings") -> (w125:T16)
              }
              event "Stop": Value Change {
                n49 = event-data() -> ()  [unwired: 1 in, 1 out]
              }
            }
          }
          frame "Generate Report" {
            n50 = stacked-sequence {
              seq-local: [w149 _] -> [_ w193]
              tunnel: w146 -> [w152 w194]
              tunnel: [w151 _] -> w145
              tunnel: w144 -> [w150 _]
              tunnel: w143 -> [_ w196]
              tunnel: [_ w195] -> w142
              tunnel: [_ w193] -> w141
              frame #0 {
                n51 = case shown="True" w150 {
                  tunnel: w152 -> [w154 w157]
                  tunnel: [w154 w156] -> w151
                  tunnel: [FALSE w155] -> w149
                  frame False {
                  }
                  frame True {
                    n52 = local read "Template Path"() -> (w160:path)
                    n53 = local read "JPEG1 Path"() -> (w159:path)
                    n54 = local read "JPEG2 Path"() -> (w158:path)
                    n55 = Build Array(w160, w159, w158) -> (w165:path[])
                    n56 = for {
                      tunnel: w165 -> [w170] mode=indexing
                      tunnel: [w167] -> w162 mode=indexing
                      shift-right: [w173] -> w164
                      shift-left: _ -> [w174]
                      n57 = Path To String(path=w170) -> (string=w171:string)
                      n58 = call <vilib>:"Check if File or Folder Exists.vi"("error in (no error)"=w174, "path"=w170) -> ("error out"=w173:errorcluster, "file or folder exists?"=w169:bool)  [unwired: 7 in, 1 out]
                      n59 = call <vilib>:"Trim Whitespace.vi"("string"=w171) -> ("trimmed string"=w172:string)  [unwired: 1 in]
                      n60 = Empty String/Path?(string/path=w172) -> (empty?=w168:bool)
                      n61 = Not(x=w168) -> (.not. x?=w166:bool)
                      n62 = And(x=w166, y=w169) -> (x .and. y?=w167:bool)
                    }
                    n63 = Boolean Array To Number(Boolean array=w162) -> (number=w161:u32)
                    n64 = And Array Elements(Boolean array=w162) -> (logical AND=w163:bool)
                    n65 = case shown="False" w163 {
                      tunnel: w157 -> [w179 w192]
                      tunnel: [w179 w191] -> w156
                      tunnel: [w180 w190] -> _
                      tunnel: w164 -> [w180 w187]
                      tunnel: w161 -> [w181 _]
                      tunnel: w160 -> [_ w186]
                      tunnel: w159 -> [_ w185]
                      tunnel: w158 -> [_ w184]
                      tunnel: [TRUE FALSE] -> w155
                      frame False {
                        n66 = Index Array(array=string[] ["Template and JPEG paths are not valid or don't exist", "JPEG paths are not valid or don't exist", "JPEG 2 & Template  paths are not valid", "JPEG 2 path is not valid", "JPEG 1 & Template  paths are not valid", "JPEG 1 path is not valid", "Template path is not valid"], index=w181) -> (element=w177:string)
                        n67 = Concatenate Strings(w177, "\n\nPlease correct the issue." ("string")) -> (w176:string)
                        n68 = One Button Dialog(message=w176) -> ()  [unwired: 1 in, 1 out]
                      }
                      frame True {
                        n69 = call "Username.vi"("error in"=w187) -> ("error out"=w190:errorcluster, "Report Store Path_Out"=w188:path, "User Name_Out"=w189:string)  [unwired: 8 in]
                        n70 = Bundle By Name(cluster=w192, "Path Settings:.Template Path"=w186, "Path Settings:.JPEG1 Path"=w185, "Path Settings:.JPEG2 Path"=w184, "User Name"=w189, "Path Settings:.Report Path"=w188) -> (w191:T16)
                      }
                    }
                  }
                }
              }
              frame #1 {
                n71 = case shown="False" w193 {
                  tunnel: w196 -> [w199 w218]
                  tunnel: [w198 w218] -> w195
                  tunnel: w194 -> [w197 _]
                  frame False {
                    n72 = flat-sequence {
                      tunnel: w199 -> [w209]
                      tunnel: [w209] -> w207
                      tunnel: [w208] -> w206
                      tunnel: w197 -> [w211]
                      tunnel: w207 -> [w213]
                      tunnel: [w212] -> w205
                      tunnel: [w210] -> w204
                      tunnel: w206 -> [w210]
                      tunnel: [w217] -> w198
                      tunnel: w205 -> [w217]
                      tunnel: w204 -> [w215]
                      tunnel: [w214] -> w202
                      frame #0 {
                        n73 = Tick Count (ms)() -> (millisecond timer value=w208:u32)
                      }
                      frame #1 {
                        n74 = call "Generate Report.vi"("Data_In"=w211, "error in"=w213) -> ("error out"=w212:errorcluster)  [unwired: 9 in]
                      }
                      frame #2 {
                        n75 = Tick Count (ms)() -> (millisecond timer value=w216:u32)
                        n76 = Subtract(x=w216, y=w215) -> (x-y=w214:u32)
                      }
                    }
                    n77 = Divide(x=w202, y=u32 1000) -> (x/y=w203:dbl)
                    n78 = To Unsigned Long Integer(number=w203) -> (unsigned 32bit integer=→"Time Taken (Seconds)":u32)
                  }
                  frame True {
                  }
                }
              }
            }
          }
          frame "Error" {
            n79 = call <vilib>:"Simple Error Handler.vi"("error in (no error)"=w222) -> ("error out"=w221:errorcluster)  [unwired: 4 in, 4 out]
            n80 = call <vilib>:"Clear Errors.vi"("error in (no error)"=w221) -> ("error out"=w220:errorcluster)  [unwired: 5 in, 1 out]
          }
          frame "Exit" {
          }
        }
      }
    }
    frame True {
      w231 = T20 1 items=["no dialog", "OK message", "continue or stop message", "OK message + warnings", "continue/stop + warnings"] ("type of dialog (OK msg:1)")
      n81 = call <vilib>:"Simple Error Handler.vi"("type of dialog (OK msg:1)"=w231, "error in (no error)"=w232) -> ()  [unwired: 3 in, 5 out]
    }
  }
  "error out" <- w4
